vi "WSVCAP SHL Host LL Interface Core Instance Manager.vi"(4 "I/O Choice (read)":T1, 6 "FPGA":T5, 8 "error in (no error)":errorcluster, 11 "FPGA Interface In":T2={"Settings"={"I2C Slave Address"=144, "I2C Clock Rate (Hz)"=20.0, "SPI Clock Rate (Hz)"=50000.0, "RFFE Slave Address"=255, "RFFE Clock Rate (Hz)"=20.0, "Simulate FPGA"=TRUE, "C1 Cap DAC Default"=165, "C2 Cap DAC Default"=165, "C3 Cap DAC Default"=134, "C4 Cap DAC Default"=150}, "FPGA Resource"="", "Online"=FALSE, "I2C Wait Ticks"=0, "SPI Wait Ticks"=0, "RFFE Wait Ticks"=0, "FPGA VI Reference (FPGA Mode)"=refnum, "FPGA VI Reference (Sim Mode)"=refnum} {"Settings"."C4 Cap DAC Default" format="0x%02x"; "Settings"."C3 Cap DAC Default" format="0x%02x"; "Settings"."C2 Cap DAC Default" format="0x%02x"; "Settings"."C1 Cap DAC Default" format="0x%02x"; "Settings"."RFFE Clock Rate (Hz)" format="%.0f Hz"; "Settings"."RFFE Slave Address" format="0x%02x"; "Settings"."I2C Clock Rate (Hz)" format="%.0f Hz"; "Settings"."SPI Clock Rate (Hz)" format="%.0f Hz"; "Settings"."I2C Slave Address" format="0x%02x"}) -> (0 "error out":errorcluster, 3 "FGPA Interface Out":T2={"Settings"={"I2C Slave Address"=144, "I2C Clock Rate (Hz)"=20.0, "SPI Clock Rate (Hz)"=50000.0, "RFFE Slave Address"=255, "RFFE Clock Rate (Hz)"=20.0, "Simulate FPGA"=TRUE, "C1 Cap DAC Default"=165, "C2 Cap DAC Default"=165, "C3 Cap DAC Default"=134, "C4 Cap DAC Default"=150}, "FPGA Resource"="", "Online"=FALSE, "I2C Wait Ticks"=0, "SPI Wait Ticks"=0, "RFFE Wait Ticks"=0, "FPGA VI Reference (FPGA Mode)"=refnum, "FPGA VI Reference (Sim Mode)"=refnum} {"Settings"."C4 Cap DAC Default" format="0x%02x"; "Settings"."C3 Cap DAC Default" format="0x%02x"; "Settings"."C2 Cap DAC Default" format="0x%02x"; "Settings"."C1 Cap DAC Default" format="0x%02x"; "Settings"."RFFE Clock Rate (Hz)" format="%.0f Hz"; "Settings"."RFFE Slave Address" format="0x%02x"; "Settings"."I2C Clock Rate (Hz)" format="%.0f Hz"; "Settings"."SPI Clock Rate (Hz)" format="%.0f Hz"; "Settings"."I2C Slave Address" format="0x%02x"})   [LabVIEW 2017]
uses:
  Type Defs/WSVCAP SHL FPGA Enum.ctl
  Type Defs/WSVCAP SHL Core System Cluster.ctl
  Type Defs/WSVCAP SHL I2C Settings Cluster.ctl
  Type Defs/WSVCAP SHL FPGA Ref.ctl
  user.lib/Utilities/Type Defs/MISC IO Choice Enum.ctl
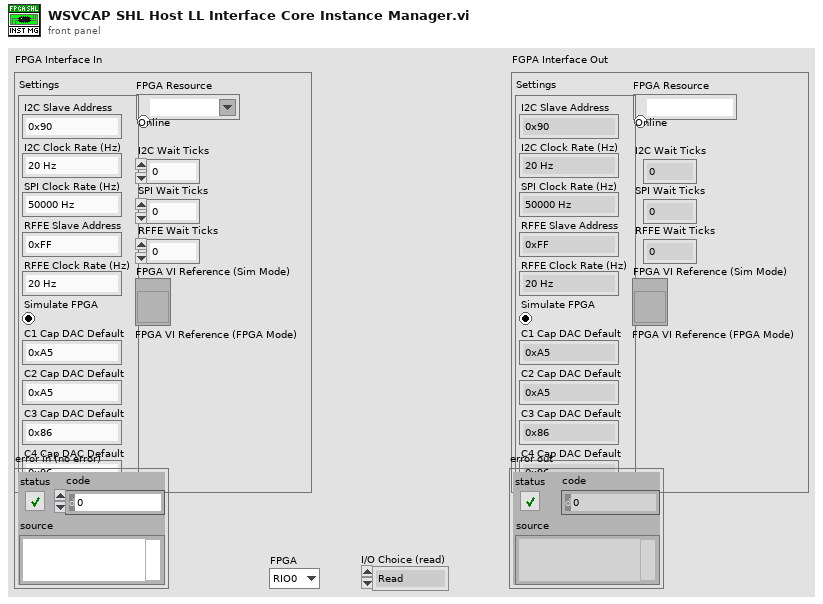
[diagram p1: front panel]
types:
  T1 = typedef "MISC IO Choice Enum.ctl" = enum16{"Read", "Write"}
  T2 = typedef "WSVCAP SHL Core System Cluster.ctl" = cluster{"Settings":T3, "FPGA Resource":tag, "Online":bool, "I2C Wait Ticks":u32, "SPI Wait Ticks":u32, "RFFE Wait Ticks":u32, "FPGA VI Reference (FPGA Mode)":T4, "FPGA VI Reference (Sim Mode)":refnum<vi>}
  T3 = typedef "WSVCAP SHL I2C Settings Cluster.ctl" = cluster{"I2C Slave Address":u8, "I2C Clock Rate (Hz)":dbl, "SPI Clock Rate (Hz)":dbl, "RFFE Slave Address":u8, "RFFE Clock Rate (Hz)":dbl, "Simulate FPGA":bool, "C1 Cap DAC Default":u8, "C2 Cap DAC Default":u8, "C3 Cap DAC Default":u8, "C4 Cap DAC Default":u8}
  T4 = typedef "WSVCAP SHL FPGA Ref.ctl" = refnum<k20>
  T5 = typedef "WSVCAP SHL FPGA Enum.ctl" = enum16{"RIO0", "RIO1"}
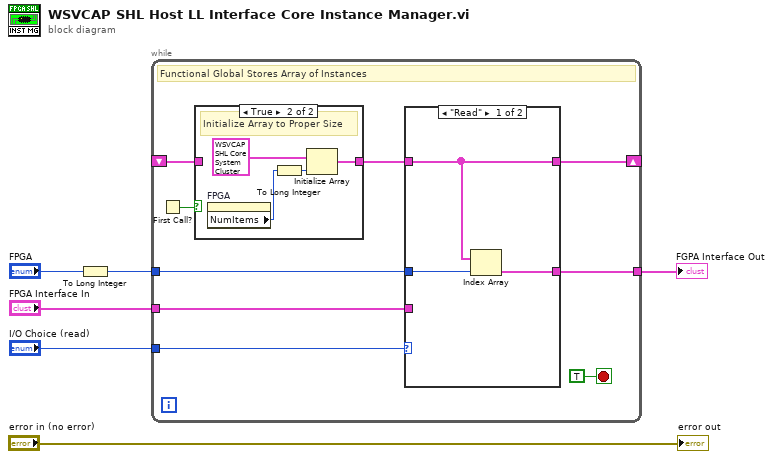
[diagram p0: block diagram]
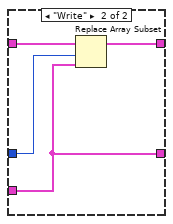
[diagram p2: hidden frame]
diagram:
  n1 = To Long Integer(number="FPGA") -> (32bit integer=w3:i32)
  n2 = while {
    shift-right: [w10] -> _
    shift-left: _ -> [w12]
    tunnel: "I/O Choice (read)" -> [w13]
    tunnel: "FPGA Interface In" -> [w9]
    tunnel: w3 -> [w8]
    tunnel: [w7] -> w2
    stop <- TRUE ("stop") stop-if-true
    # "Functional Global Stores Array of Instances"
    n3 = First Call?() -> (First Call?: T/F=w15:bool)
    n4 = case shown="True" w15 {
      tunnel: w12 -> [w23 _]
      tunnel: [w23 w25] -> w11
      frame False {
        # "Use Stored Instances"
      }
      frame True {
        # "Initialize Array to Proper Size"
        n5 = property on="FPGA" class="Enum (strict)"() -> ("NumItems"=w27:u32)  [unwired: 2 in, 2 out]
        n6 = To Long Integer(number=w27) -> (32bit integer=w26:i32)
        n7 = Initialize Array(T2 {"Settings"={"I2C Slave Address"=144, "I2C Clock Rate (Hz)"=20.0, "SPI Clock Rate (Hz)"=50000.0, "RFFE Slave Address"=255, "RFFE Clock Rate (Hz)"=20.0, "Simulate FPGA"=TRUE, "C1 Cap DAC Default"=165, "C2 Cap DAC Default"=165, "C3 Cap DAC Default"=134, "C4 Cap DAC Default"=150}, "FPGA Resource"="", "Online"=FALSE, "I2C Wait Ticks"=0, "SPI Wait Ticks"=0, "RFFE Wait Ticks"=0, "FPGA VI Reference (FPGA Mode)"=refnum, "FPGA VI Reference (Sim Mode)"=refnum} ("FGPA Interface Out"), w26) -> (w25:T2[])
      }
    }
    n8 = case shown="\"Read\"" w13 {
      tunnel: [w16 w21] -> w10
      tunnel: w11 -> [w16 w22]
      tunnel: w9 -> [_ w19]
      tunnel: w8 -> [w18 w20]
      tunnel: [w17 w19] -> w7
      frame "Read" {
        n9 = Index Array(array=w16, index=w18) -> (element=w17:T2)
      }
      frame "Write" {
        n10 = Replace Array Subset(array=w22, new element=w19, index=w20) -> (w21:T2[])
      }
    }
  }
  "FGPA Interface Out" <- w2
  "error out" <- "error in (no error)"
